vi "SetTrigger.vi"(6 "Legacy (f)?":bool, 8 "error in (no error)":errorcluster) -> (0 "error out":errorcluster)   [LabVIEW 2011]
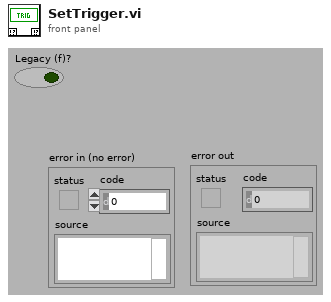
[diagram p1: front panel]
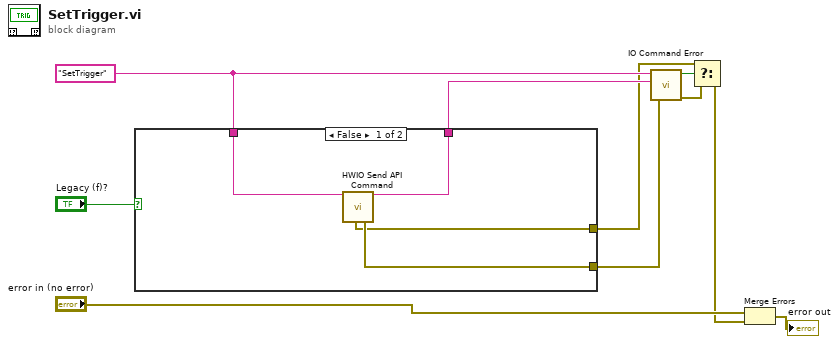
[diagram p0: block diagram]
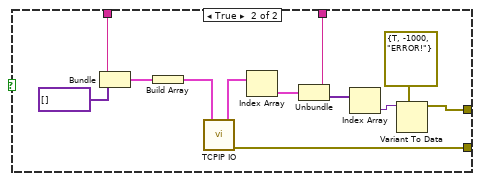
[diagram p2: hidden frame]
diagram:
  w9 = "SetTrigger"
  n1 = case shown="False" "Legacy (f)?" {
    tunnel: [w14 w24] -> w10
    tunnel: w9 -> [w12 w23]
    tunnel: [w13 w19] -> w8
    tunnel: [w11 w15] -> w2
    frame False {
      n2 = call "HWIO Send API Command.vi"("Action"=w12) -> ("Action out"=w13:string, "HWError"=w11:errorcluster, "error out"=w14:errorcluster)  [unwired: 7 in, 5 out]
    }
    frame True {
      n3 = Bundle(w23, variant[] []) -> (w25:cluster{string, variant[]})  [unwired: 1 out]
      n4 = Build Array(w25) -> (w22:cluster{string, variant[]}[])
      n5 = call "TCPIP IO.vi"("Commands"=w22) -> ("error out"=w24:errorcluster, "Responses"=w20:cluster{string, variant[]}[])  [unwired: 2 in, 3 out]
      n6 = Index Array(array=w20) -> (element=w21:cluster{string, variant[]})  [unwired: 1 in]
      n7 = Unbundle(w21) -> (w19:string, w16:variant[])
      n8 = Index Array(array=w16) -> (element=w18:variant)  [unwired: 1 in]
      n9 = Variant To Data(type=errorcluster {"status"=TRUE, "code"=-1000, "source"="ERROR!"} ("error out"), Variant=w18) -> (data=w15:errorcluster)  [unwired: 1 in, 1 out]
    }
  }
  n10 = call "IO Command Error.vi"("error in (no error)"=w10, "Command Returned (\"\")"=w8, "Command Sent (\"\")"=w9) -> ("error out"=w4:errorcluster, "HW ERR?"=w5:bool)  [unwired: 3 out]
  n11 = Select(t=w2, s=w5, f=w4) -> (s? t:f=w3:errorcluster)
  n12 = Merge Errors("error in (no error)", w3) -> (→"error out":errorcluster)
